vi "Reshape2.vi"(6 "Numeric":i32, 9 "EEG_Channel_Num":i32, 10 "all rows":dbl[][](array[numeric]), 11 "Numeric 2":dbl) -> (3 "Array":dbl[][](array[numeric]))   [LabVIEW 2014]
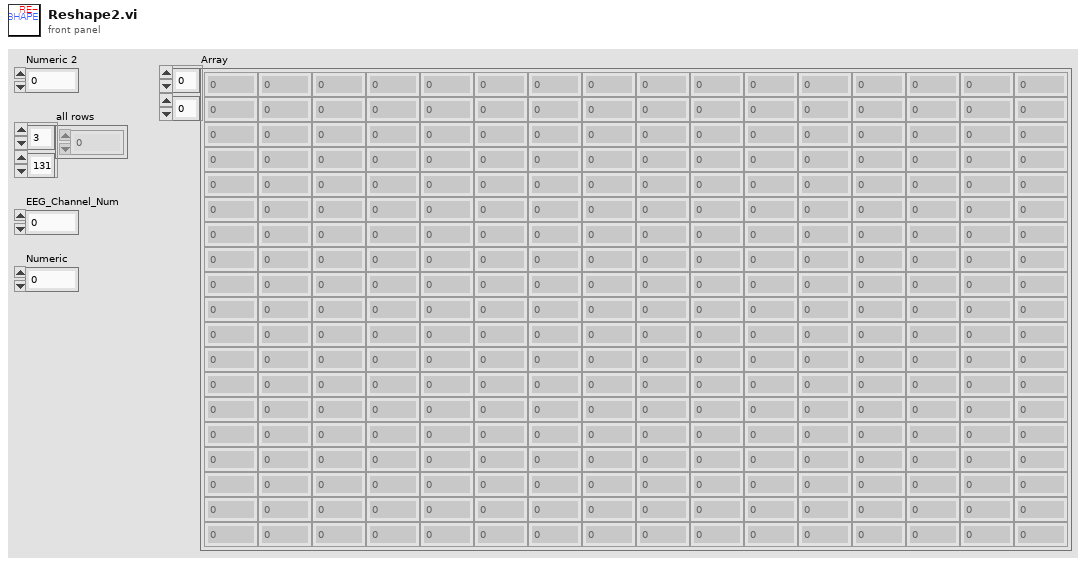
[diagram p1: front panel]
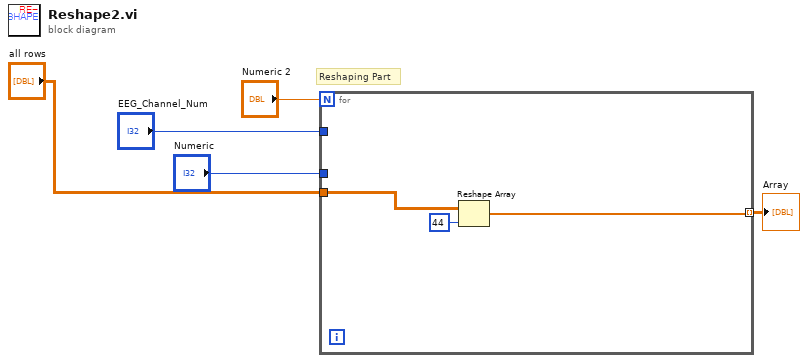
[diagram p0: block diagram]
diagram:
  # "Reshaping Part"
  n1 = for {
    N: "Numeric 2" -> [_]
    tunnel: "EEG_Channel_Num" -> [_]
    tunnel: "all rows" -> [w7]
    tunnel: "Numeric" -> [_]
    tunnel: [w8] -> w5 mode=indexing
    n2 = Reshape Array(w7, 44 ("dimension size")) -> (w8:dbl[])
  }
  "Array" <- w5
